vi "Close Device.vi"(8 "error in (no error)":errorcluster, 11 "HRF_Device":refnum<class "HRF_Device.lvclass">) -> (0 "error out":errorcluster)   [LabVIEW 2020, in "HRF_Device.lvclass"]
uses:
  HRF_Device.lvclass
  HRF_Device.lvclass/HRF_Device.ctl
  D:/work/HackRF/Labview Driver/NetHackrf.dll
  NetHackrf.dll
panel:
  out "error out 2":errorcluster
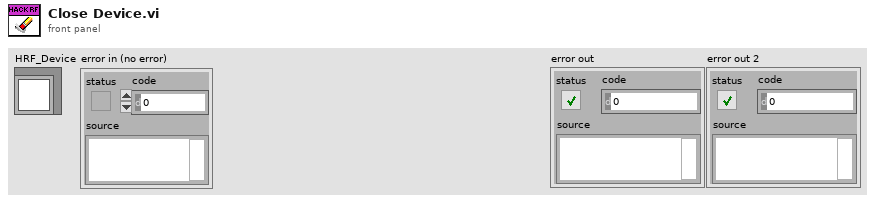
[diagram p1: front panel]
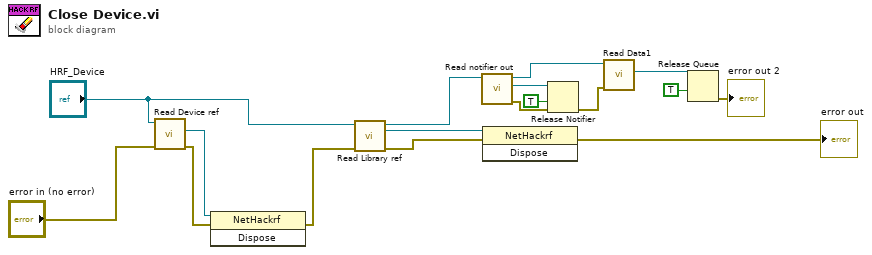
[diagram p0: block diagram]
diagram:
  n1 = call "Read Device ref.vi"("error in (no error)"="error in (no error)", "HRF_Device in"="HRF_Device") -> ("error out"=w10:errorcluster, "Device ref"=w16:refnum<k24>)  [unwired: 7 in, 1 out]
  n2 = invoke class="NetHackrf" method="Dispose"(reference=w16, error in=w10) -> (error out=w15:errorcluster)  [unwired: 1 in, 2 out]
  n3 = call "Read Library ref.vi"("error in (no error)"=w15, "HRF_Device in"="HRF_Device") -> ("error out"=w13:errorcluster, "Library ref"=w14:refnum<k24>, "HRF_Device out"=w9:refnum<class "HRF_Device.lvclass">)  [unwired: 7 in]
  n4 = call "Read notifier out.vi"("HRF_Device in"=w9) -> ("error out"=w7:errorcluster, "notifier out"=w8:refnum<notifier>, "HRF_Device out"=w2:refnum<class "HRF_Device.lvclass">)  [unwired: 8 in]
  n5 = invoke class="NetHackrf" method="Dispose"(reference=w14, error in=w13) -> (error out=→"error out":errorcluster)  [unwired: 1 in, 2 out]
  n6 = Release Notifier(notifier=w8, force destroy? (F)=TRUE, error in (no error)=w7) -> (error out=w3:errorcluster)  [unwired: 2 out]
  n7 = call "Read Data1.vi"("error in (no error)"=w3, "HRF_Device in"=w2) -> ("Data"=w1:refnum<queue>)  [unwired: 7 in, 2 out]
  n8 = Release Queue(queue=w1, force destroy? (F)=TRUE) -> (error out=→"error out 2":errorcluster)  [unwired: 1 in, 2 out]
